vi "Comprobar Temperatura Correcta.vi"(2 "Temp.Min IN":dbl, 3 "Temp.Max  IN":dbl) -> (0 "Temp.Min OUT":dbl, 1 "Temp.Max OUT":dbl)   [LabVIEW 2021]
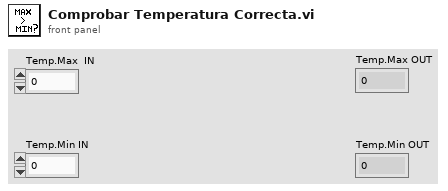
[diagram p1: front panel]
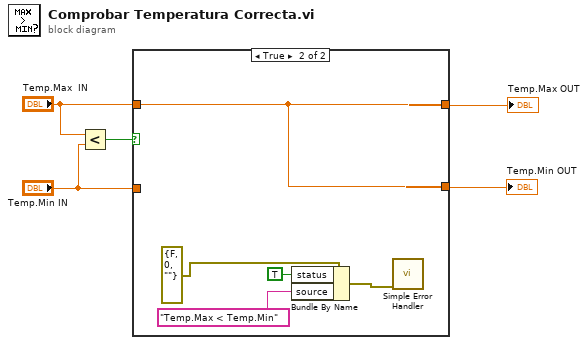
[diagram p0: block diagram]
diagram:
  n1 = Less?(x="Temp.Max  IN", y="Temp.Min IN") -> (x < y?=w5:bool)
  n2 = case shown="True" w5 {
    tunnel: [w7 w12] -> w2
    tunnel: "Temp.Max  IN" -> [w7 w12]
    tunnel: [w6 w12] -> w1
    tunnel: "Temp.Min IN" -> [w6 _]
    frame False {
    }
    frame True {
      n3 = Bundle By Name(cluster=errorcluster {"status"=FALSE, "code"=0, "source"=""} ("error constant"), "status"=TRUE, "source"="Temp.Max < Temp.Min") -> (w11:errorcluster)
      n4 = call <vilib>:"Simple Error Handler.vi"("error in (no error)"=w11) -> ()  [unwired: 4 in, 5 out]
    }
  }
  "Temp.Max OUT" <- w2
  "Temp.Min OUT" <- w1
